vi "Actor Core.vi"(8 "error in":errorcluster, 11 "Car Wash Controller in":refnum<class "Sim Entry Console Actor.lvclass">) -> (0 "error out":errorcluster, 3 "Actor out":refnum<class "Actor.lvclass">)   [LabVIEW 2019, in "Sim Entry Console Actor.lvlib" / "Sim Entry Console Actor.lvclass"]
doc: "(<B>Filename</B>: Actor Framework.lvlib:Actor.lvclass:Actor Core.vi)\n\nReceives messages to the actor, reacts to them, and initiates any error handling that may shut the actor down.\n\nDescendant classes may override this VI to append parallel tasks for the actor to complete while it handles messages. Overrides use the Call Parent Method node."
uses:
  Sim Entry Console Actor.lvclass
  <vilib>/ActorFramework/Stop Msg/Stop Msg.lvclass
  <vilib>/ActorFramework/Actor/Actor.lvclass
  Entry Console Actor/Entry Console Actor/Entry Console Actor.lvclass
  C:/Workspace/CLA/Carwasher AF 2nd/Entry Console Actor/Entry Console Actor/Entry Console Actor.lvclass
  C:/Program Files (x86)/National Instruments/LabVIEW 2019/vi.lib/ActorFramework/Actor/Actor.lvclass
  Sim Entry Console Actor Messages/Enable Wash Steps Msg/Enable Wash Steps Msg.lvclass
  Car Wash Controller/Car Wash Controller Messages/Set Wash Steps Msg/Set Wash Steps Msg.lvclass
  Car Wash Controller/Car Wash Controller Messages/Set State Msg/Set State Msg.lvclass
  Car Wash Controller/Car Wash Controller/States -Enum.ctl
  Car Wash Controller/Car Wash Controller/Car Wash Controller.lvclass
  Car Wash Controller/Car Wash Controller/Wash Steps.ctl
panel:
  in  "Start":bool
  in  "Wash Steps":T1
  # "UI1"
  # "UI2\nUI2A\nUI2A1\nUI2A2"
  # "Mechanical Switch type"
  # "UI2B\nUI2B1"
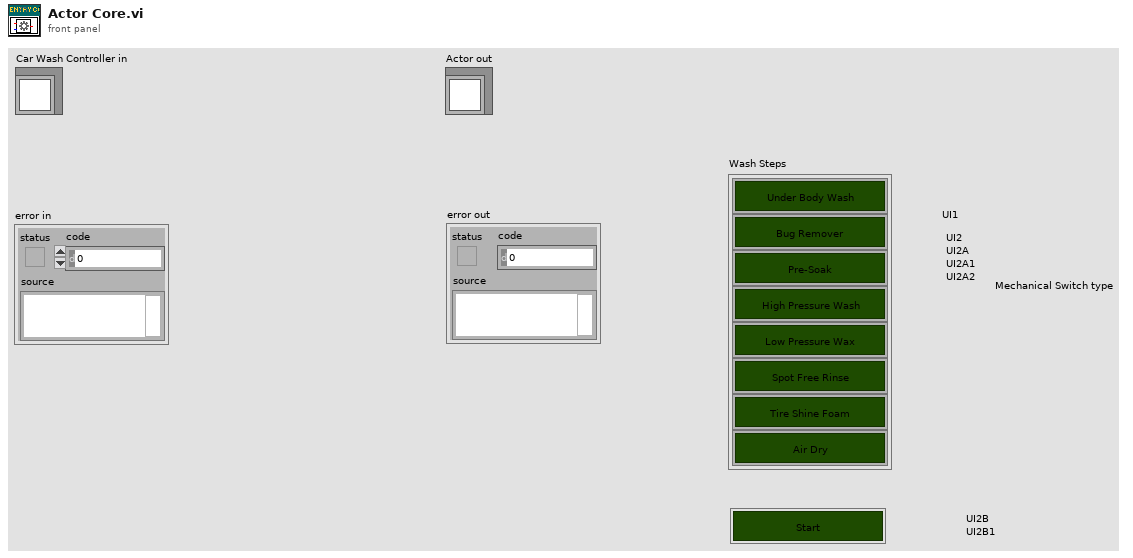
[diagram p1: front panel]
types:
  T1 = typedef "Car Wash Controller.lvlib/Car Wash Controller.lvclass/Wash Steps.ctl" = cluster{"Under Body Wash":bool, "Bug Remover":bool, "Pre-Soak":bool, "High Pressure Wash (Default)":bool, "Low Pressure Wax":bool, "Spot Free Rinse":bool, "Tire Shine Foam":bool, "Air Dry":bool}
  T2 = typedef "Car Wash Controller.lvlib/Car Wash Controller.lvclass/States -Enum.ctl" = enum16{"Inital", "Wait for Start", "Start", "Wait for Vehicle Position", "Wash Step Execution", "Wash Step/Cycle Completion", "Wash Exit", "Wash Abort/Terminate State"}
  T3 = enum8{"Enabled", "Disabled", "Disabled and Grayed Out"}
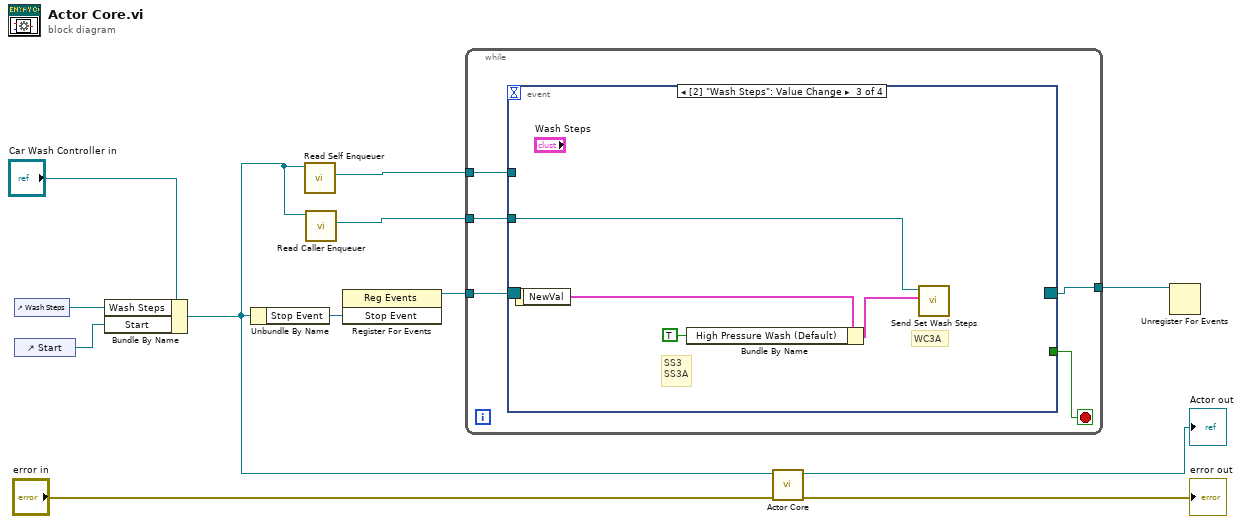
[diagram p0: block diagram]
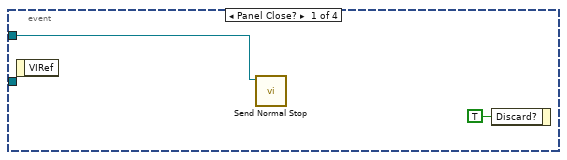
[diagram p2: hidden frame]
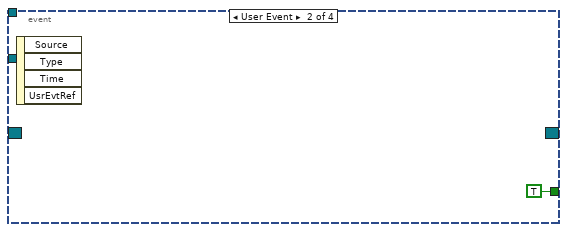
[diagram p3: hidden frame]
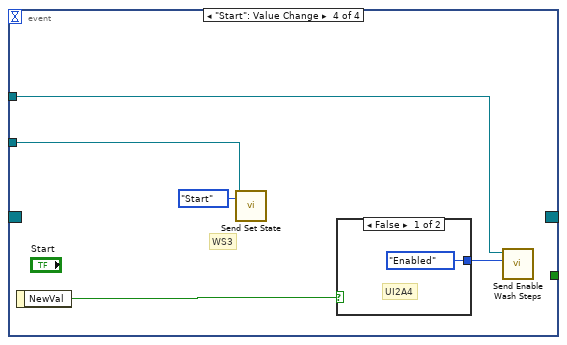
[diagram p4: hidden frame]
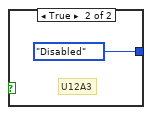
[diagram p5: hidden frame]
diagram:
  n1 = control-ref of="Wash Steps"() -> (w4:refnum<vi>)
  n2 = control-ref of="Start"() -> (w3:refnum<vi>)
  n3 = Bundle By Name(cluster="Car Wash Controller in", "Wash Steps"=w4, "Start"=w3) -> (w2:refnum<class "Sim Entry Console Actor.lvclass">)
  n4 = Unbundle By Name(w2) -> ("Stop Event"=w6:refnum<user-event>)
  n5 = call <vilib>:"Read Self Enqueuer.vi"("Actor"=w2) -> ("Self Enqueuer"=w7:refnum<class "Message Enqueuer.lvclass">)  [unwired: 10 in]
  n6 = call <vilib>:"Read Caller Enqueuer.vi"("Actor"=w2) -> ("Caller Enqueuer"=w1:refnum<class "Message Enqueuer.lvclass">)  [unwired: 10 in]
  n7 = register-events(w6) -> (reference out=w9:refnum<event-registration>)  [unwired: 2 in, 1 out]
  n8 = while {
    tunnel: w9 -> [w16]
    tunnel: [w15] -> w8
    tunnel: w7 -> [w14]
    tunnel: w1 -> [w13]
    stop <- w17 stop-if-true
    n9 = event shown="[2] \"Wash Steps\": Value Change" {
      selector: w16 -> [_ _ _ _]
      dyn-events: [_ _ _ _] -> w15
      timeout: _ -> [_ _ _ _]
      tunnel: [_ TRUE _ _] -> w17
      tunnel: w14 -> [w18 _ _ w27]
      tunnel: w13 -> [_ _ w24 w26]
      event Panel Close? {
        n10 = event-data() -> ()  [unwired: 1 in, 1 out]
        n11 = call <vilib>:"Send Normal Stop.vi"("Message Enqueuer"=w18) -> ()  [unwired: 10 in, 1 out]
        n12 = event-data("Discard?"=TRUE) -> ()  [unwired: 1 in, 1 out]
      }
      event User Event {
        n13 = event-data() -> ()  [unwired: 1 in, 4 out]
      }
      event Value Change {
        # "WC3A"
        # "SS3\nSS3A"
        n14 = event-data() -> ("NewVal"=w23:T1)  [unwired: 1 in]
        n15 = Bundle By Name(cluster=w23, "High Pressure Wash (Default)"=TRUE) -> (w21:T1)
        n16 = call "Send Set Wash Steps.vi"("Wash Steps"=w21, "Message Enqueuer"=w24) -> ()  [unwired: 8 in, 2 out]
      }
      event "Start": Value Change {
        # "WS3"
        n17 = event-data() -> ("NewVal"=w29:bool)  [unwired: 1 in]
        n18 = call "Send Set State.vi"("State"=States_-Enum."Start", "Message Enqueuer"=w26) -> ()  [unwired: 8 in, 2 out]
        n19 = case shown="False" w29 {
          tunnel: [T3."Enabled" ("Disabled") T3."Disabled" ("Disabled")] -> w28
          frame False {
            # "UI2A4"
          }
          frame True {
            # "U12A3"
          }
        }
        n20 = call "Send Enable Wash Steps.vi"("Disabled"=w28, "Message Enqueuer"=w27) -> ()  [unwired: 8 in, 2 out]
      }
    }
  }
  n21 = call-parent "Actor Core.vi"("error in"="error in", "Actor in"=w2) -> ("error out"=→"error out":errorcluster, "Actor out"=→"Actor out":refnum<class "Actor.lvclass">)  [unwired: 8 in]
  n22 = Unregister For Events(event registration refnum=w8) -> ()  [unwired: 1 in, 1 out]
